vi "GetValue.vi"(8 "error in":errorcluster, 11 "StringMeasure in":refnum<class "StringMeasure.lvclass">) -> (0 "error out":errorcluster, 2 "Value":string, 3 "StringMeasure out":refnum<class "StringMeasure.lvclass">)   [LabVIEW 2021, in "ProligentXMLGenerator.lvlib" / "StringMeasure.lvclass"]
doc: "Defines the value acquired by the measure."
uses:
  StringMeasure.lvclass
  StringMeasure.lvclass/StringMeasure.ctl
  Base/String_4000/String_4000.lvclass
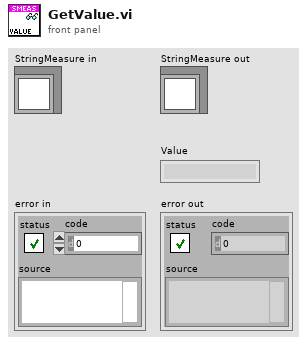
[diagram p1: front panel]
types:
  T1 = typedef "ProligentXMLGenerator.lvlib/StringMeasure.lvclass/Data.ctl" = cluster{"Value":refnum<class "String_4000.lvclass">}
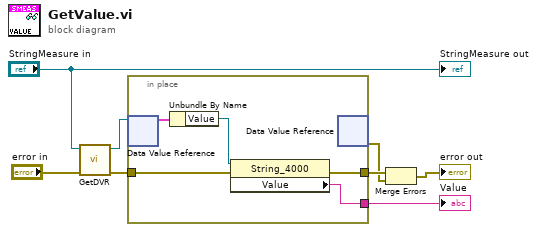
[diagram p0: block diagram]
diagram:
  n1 = call "GetDVR.vi"("error in"="error in", "StringMeasure"="StringMeasure in") -> ("error out"=w4:errorcluster, "DVRReference"=w2:refnum<data-value>)  [unwired: 8 in]
  n2 = in-place "In Place Element Structure" {
    in-place-border: [w9] -> w1
    in-place-border: w4 -> [w11]
    in-place-border: [w10] -> w6
    n3 = in-place-dvr #1(w2) -> (w13:T1)  [unwired: 1 out]
    n4 = Unbundle By Name(w13) -> ("Value"=w12:refnum<class "String_4000.lvclass">)
    n5 = property class="String_4000"(reference=w12, error in=w11) -> (error out=w10:errorcluster, "Value"=w9:string)  [unwired: 1 out]
    n6 = in-place-dvr #1() -> (w5:errorcluster)  [unwired: 1 in, 1 out]
  }
  "Value" <- w1
  n7 = Merge Errors(w6, w5) -> (→"error out":errorcluster)
  "StringMeasure out" <- "StringMeasure in"
